vi "PID_controller_03.vi"() -> ()   [LabVIEW 2011]
uses:
  <vilib>/Platform/TimedLoop/XDataNode/nitl_modes.ctl
  <vilib>/Platform/TimedLoop/XDataNode/timing_clust.ctl
  <vilib>/Platform/TimedLoop/XDataNode/wakeup.ctl
  <vilib>/Platform/TimedLoop/XDataNode/XDataNode.xnode
  <vilib>/Platform/TimedLoop/XDataNode/XDNodeRunTimeDep.lvlib
panel:
  out "S00":dbl
  out "S10":dbl
  out "S20":dbl
  out "S11":dbl
  out "S01":dbl
  out "weight":dbl[](array[numeric])
  in  "# of points to watch":i32
  in  "alpha":dbl=-1.0
  out "t0":dbl
  out "error(t)":cluster{dbl, "Value":dbl}[](array[cluster])
  out "error out":errorcluster
  out "first":bool=TRUE
  out "P (torr)":string
  out "XY Graph":T1(graph)
  out "current value":dbl
  in  "stop":bool
  in  "Period (s)":dbl
  out "Process value":dbl
  out "derivative":dbl
  out "integral":dbl
  out "error":dbl
  out "Current angle (deg)":dbl
  in  "Kd":dbl
  in  "Ki":dbl
  in  "Kp":dbl
  out "Current P (torr)":dbl
  in  "Set Point (torr)":dbl
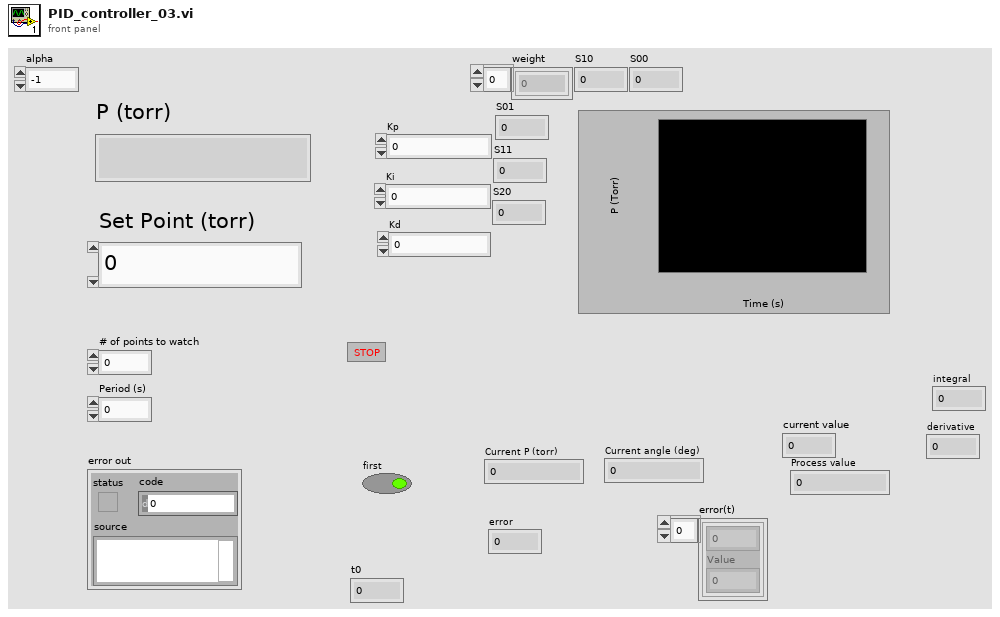
[diagram p1: front panel]
types:
  T1 = cluster{"Value":cluster{"element":dbl, "element":dbl}[]}[]
  T2 = typedef "XDNodeRunTimeDep.lvlib/nitl_modes.ctl" = enum32{"No Change", "Process missed periods, maintain original phase", "Discard missed periods, maintain original phase", "Process missed periods, ignore original phase", "Discard missed periods, ignore original phase"}
  T3 = typedef "XDNodeRunTimeDep.lvlib/timing_clust.ctl" = cluster{"Expected End [f-1]":u64, "Actual End [f-1]":u64, "Finished Late? [f-1]":bool, "Expected End [i-1]":u64, "Actual End [i-1]":u64, "Finished Late? [i-1]":bool, "Expected Start [i]":u64, "Actual Start [i]":u64, "Expected Start [f]":u64, "Actual Start [f]":u64, "Source Name":string, "Structure Name":string, "Period":i64, "Deadline":i64, "Offset":i64, "Start":i64, "Priority":i32, "Timeout":i32, "Mode":T2, "Wakeup Reason":T4, "Error":errorcluster, "Source Type":string, "Secondary Source Type":string, "Global End Time":u64, "Global Start Time":u64, "Frame Duration":u64, "Iteration Duration":u64, "Assigned CPU":i32, "I/O Scan Engine Mode":u32}
  T4 = typedef "XDNodeRunTimeDep.lvlib/wakeup.ctl" = enum32{"Normal", "Aborted", "Asynchronous wakeup", "Timing source error", "Timed loop error", "Timeout"}
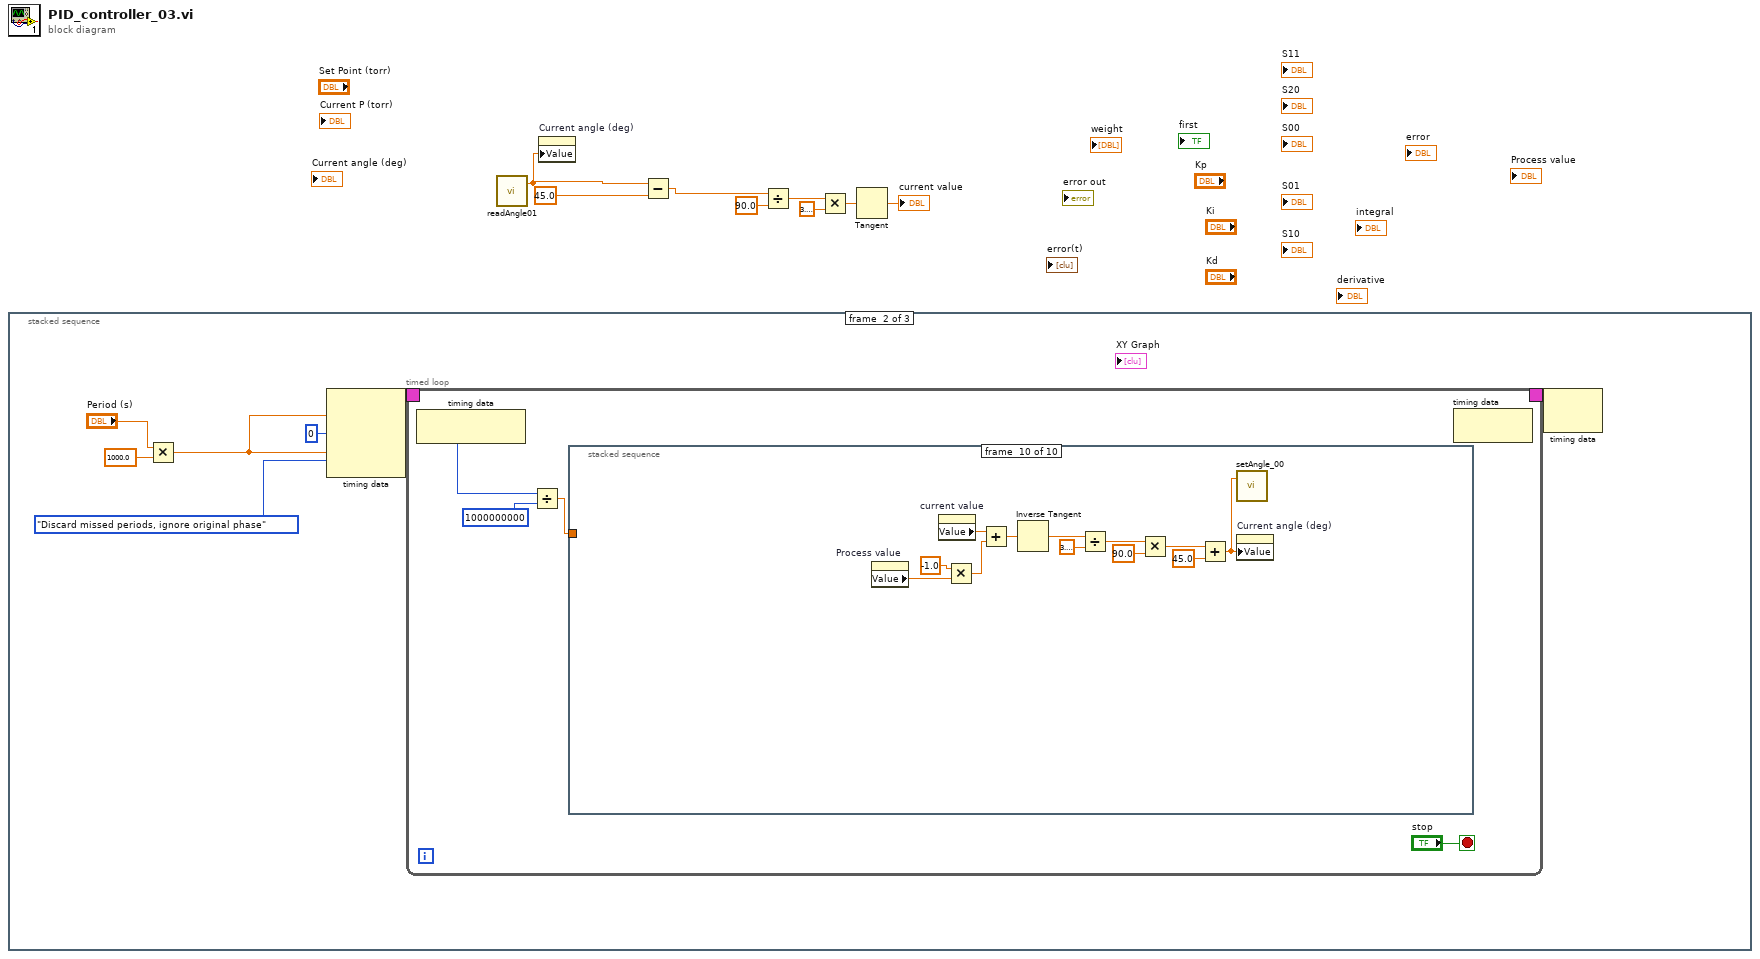
[diagram p0: block diagram]
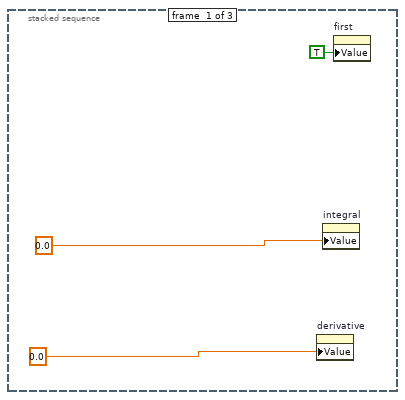
[diagram p2: hidden frame]
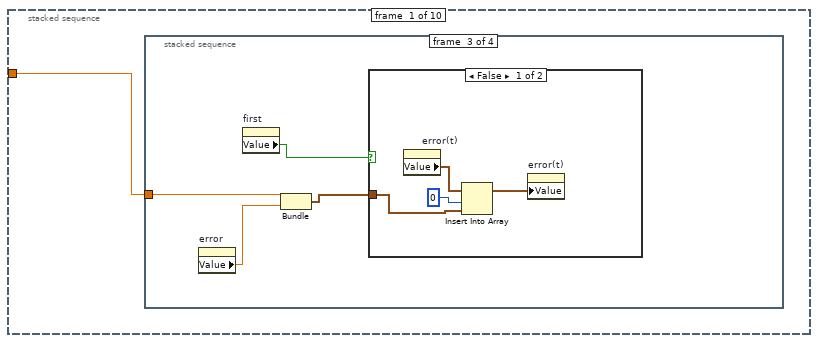
[diagram p3: hidden frame]
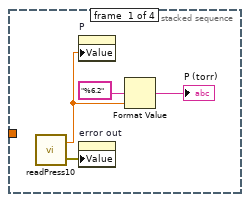
[diagram p4: hidden frame]
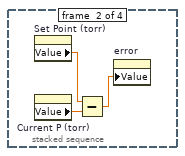
[diagram p5: hidden frame]
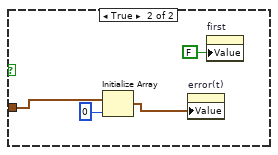
[diagram p6: hidden frame]
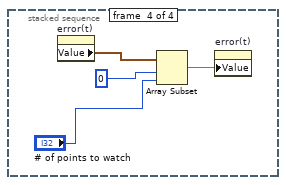
[diagram p7: hidden frame]
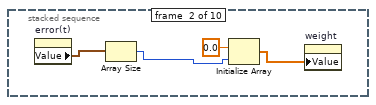
[diagram p8: hidden frame]
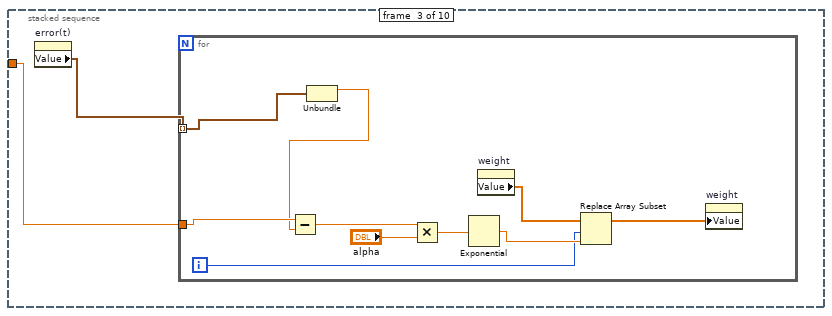
[diagram p9: hidden frame]
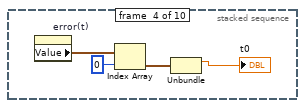
[diagram p10: hidden frame]
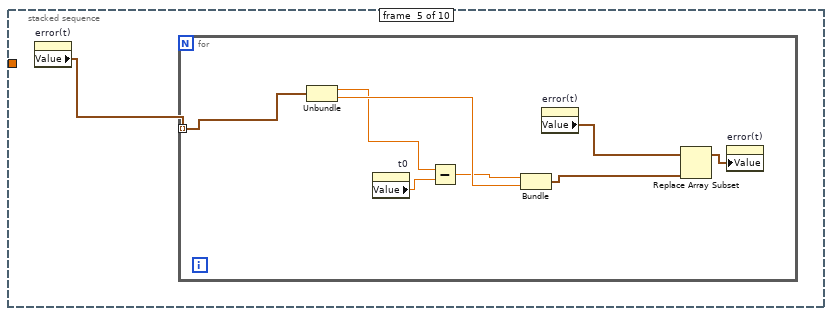
[diagram p11: hidden frame]
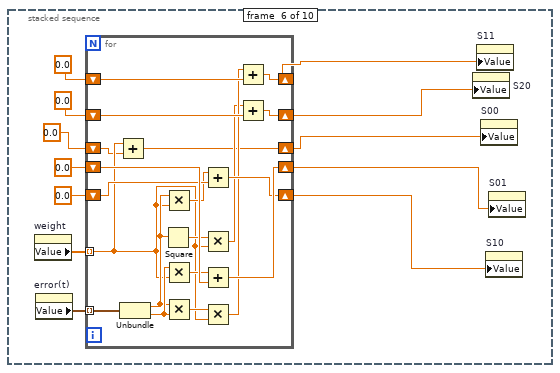
[diagram p12: hidden frame]
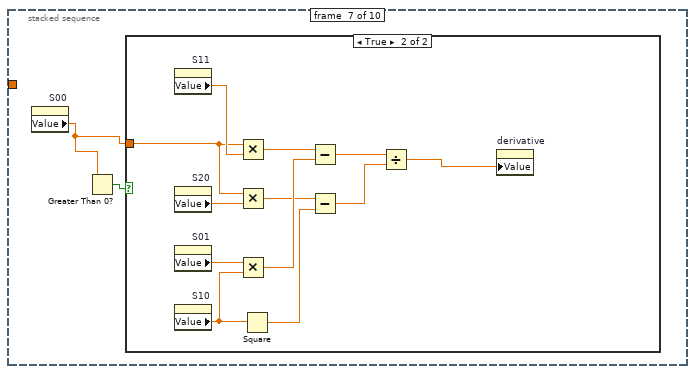
[diagram p13: hidden frame]
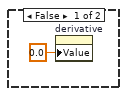
[diagram p14: hidden frame]
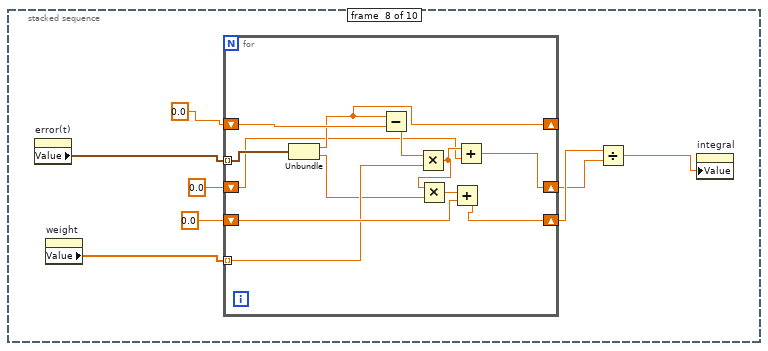
[diagram p15: hidden frame]
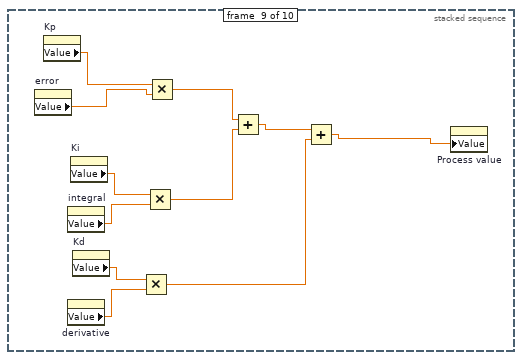
[diagram p16: hidden frame]
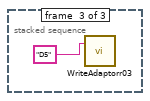
[diagram p17: hidden frame]
diagram:
  n1 = stacked-sequence {
    frame #0 {
      n2 = property on="derivative" class="DigNum (strict)"("Value"=0.0 ("derivative")) -> ()  [unwired: 2 in, 2 out]
      n3 = property on="integral" class="DigNum (strict)"("Value"=0.0 ("integral")) -> ()  [unwired: 2 in, 2 out]
      n4 = property on="first" class="Bool (strict)"("Value"=TRUE ("first")) -> ()  [unwired: 2 in, 2 out]
    }
    frame #1 {
      n5 = Multiply(x="Period (s)", y=1000.0) -> (x*y=w13:dbl)
      n6 = node-c288(w13, i64 0 ("Offset"), w13, nitl_modes."Discard missed periods, ignore original phase" ("Mode")) -> (w18:T3)
      n7 = timed-loop {
        timing: w18 -> [_]
        timing-out: [_] -> w17
        stop <- "stop" stop-if-true
        n8 = node-c288() -> (w21:i64)  [unwired: 1 in]
        n9 = Divide(x=w21, y=i64 1000000000) -> (x/y=w19:dbl)
        n10 = stacked-sequence {
          tunnel: w19 -> [w23 _ w51 _ _ _ _ _ _ _]
          frame #0 {
            n11 = stacked-sequence {
              tunnel: w23 -> [_ _ w33 _]
              frame #0 {
                n12 = call "readPress10.vi"() -> ("P"=w26:dbl, "error out"=w24:errorcluster)  [unwired: 1 in]
                n13 = property on="P" class="DigNum (strict)"("Value"=w26) -> ()  [unwired: 2 in, 2 out]
                n14 = property on="error out" class="Clust (strict)"("Value"=w24) -> ()  [unwired: 2 in, 2 out]
                n15 = Format Value(format string="%6.2", value (0)=w26) -> (output string=→"P (torr)":string)  [unwired: 1 in]
              }
              frame #1 {
                n16 = property on="Set Point (torr)" class="DigNum (strict)"() -> ("Value"=w29:dbl)  [unwired: 2 in, 2 out]
                n17 = property on="Current P (torr)" class="DigNum (strict)"() -> ("Value"=w30:dbl)  [unwired: 2 in, 2 out]
                n18 = Subtract(x=w29, y=w30) -> (x-y=w28:dbl)
                n19 = property on="error" class="DigNum (strict)"("Value"=w28) -> ()  [unwired: 2 in, 2 out]
              }
              frame #2 {
                n20 = property on="error" class="DigNum (strict)"() -> ("Value"=w32:dbl)  [unwired: 2 in, 2 out]
                n21 = property on="first" class="Bool (strict)"() -> ("Value"=w34:bool)  [unwired: 2 in, 2 out]
                n22 = Bundle(w33, "Value"=w32) -> (w31:cluster{dbl, "Value":dbl})  [unwired: 1 in]
                n23 = case shown="False" w34 {
                  tunnel: w31 -> [w35 w41]
                  frame False {
                    n24 = property on="error(t)" class="Arr (strict)"() -> ("Value"=w36:cluster{dbl, "Value":dbl}[])  [unwired: 2 in, 2 out]
                    n25 = Insert Into Array(array=w36, index=0, new element=w35) -> (w38:cluster{dbl, "Value":dbl}[])
                    n26 = property on="error(t)" class="Arr (strict)"("Value"=w38) -> ()  [unwired: 2 in, 2 out]
                  }
                  frame True {
                    n27 = Initialize Array(w41, 0 ("dimension size")) -> (w39:cluster{dbl, "Value":dbl}[])
                    n28 = property on="error(t)" class="Arr (strict)"("Value"=w39) -> ()  [unwired: 2 in, 2 out]
                    n29 = property on="first" class="Bool (strict)"("Value"=FALSE ("first")) -> ()  [unwired: 2 in, 2 out]
                  }
                }
              }
              frame #3 {
                n30 = property on="error(t)" class="Arr (strict)"() -> ("Value"=w44:cluster{dbl, "Value":dbl}[])  [unwired: 2 in, 2 out]
                n31 = Array Subset(array=w44, index=0, length="# of points to watch") -> (w46:cluster{dbl, "Value":dbl}[])
                n32 = property on="error(t)" class="Arr (strict)"("Value"=w46) -> ()  [unwired: 2 in, 2 out]
              }
            }
          }
          frame #1 {
            n33 = property on="error(t)" class="Arr (strict)"() -> ("Value"=w50:cluster{dbl, "Value":dbl}[])  [unwired: 2 in, 2 out]
            n34 = Array Size(array=w50) -> (size(s)=w48:i32)
            n35 = Initialize Array(0.0 ("element"), w48) -> (w47:dbl[])
            n36 = property on="weight" class="Arr (strict)"("Value"=w47) -> ()  [unwired: 2 in, 2 out]
          }
          frame #2 {
            n37 = property on="error(t)" class="Arr (strict)"() -> ("Value"=w52:cluster{dbl, "Value":dbl}[])  [unwired: 2 in, 2 out]
            n38 = for {
              tunnel: w52 -> [w62] mode=indexing
              tunnel: w51 -> [w59]
              i -> [w54]
              n39 = Unbundle(w62) -> (w58:dbl)  [unwired: 1 out]
              n40 = Subtract(x=w59, y=w58) -> (x-y=w57:dbl)
              n41 = Multiply(x=w57, y="alpha") -> (x*y=w60:dbl)
              n42 = Exponential(1:w60) -> (0:w56:dbl)
              n43 = property on="weight" class="Arr (strict)"() -> ("Value"=w55:dbl[])  [unwired: 2 in, 2 out]
              n44 = Replace Array Subset(array=w55, new element=w56, index=w54) -> (w53:dbl[])
              n45 = property on="weight" class="Arr (strict)"("Value"=w53) -> ()  [unwired: 2 in, 2 out]
            }
          }
          frame #3 {
            n46 = property on="error(t)" class="Arr (strict)"() -> ("Value"=w66:cluster{dbl, "Value":dbl}[])  [unwired: 2 in, 2 out]
            n47 = Index Array(array=w66, index=0) -> (element=w64:cluster{dbl, "Value":dbl})
            n48 = Unbundle(w64) -> (→"t0":dbl)  [unwired: 1 out]
          }
          frame #4 {
            n49 = property on="error(t)" class="Arr (strict)"() -> ("Value"=w67:cluster{dbl, "Value":dbl}[])  [unwired: 2 in, 2 out]
            n50 = for {
              tunnel: w67 -> [w72] mode=indexing
              n51 = Unbundle(w72) -> (w69:dbl, "Value"=w74:dbl)
              n52 = property on="t0" class="DigNum (strict)"() -> ("Value"=w75:dbl)  [unwired: 2 in, 2 out]
              n53 = Subtract(x=w69, y=w75) -> (x-y=w70:dbl)
              n54 = Bundle(w70, "Value"=w74) -> (w68:cluster{dbl, "Value":dbl})  [unwired: 1 in]
              n55 = property on="error(t)" class="Arr (strict)"() -> ("Value"=w73:cluster{dbl, "Value":dbl}[])  [unwired: 2 in, 2 out]
              n56 = Replace Array Subset(array=w73, new element=w68) -> (w71:cluster{dbl, "Value":dbl}[])  [unwired: 1 in]
              n57 = property on="error(t)" class="Arr (strict)"("Value"=w71) -> ()  [unwired: 2 in, 2 out]
            }
          }
          frame #5 {
            n58 = property on="weight" class="Arr (strict)"() -> ("Value"=w82:dbl[])  [unwired: 2 in, 2 out]
            n59 = property on="error(t)" class="Arr (strict)"() -> ("Value"=w87:cluster{dbl, "Value":dbl}[])  [unwired: 2 in, 2 out]
            n60 = for {
              tunnel: w87 -> [w103] mode=indexing
              shift-right: [w104] -> w77
              shift-left: 0.0 -> [w107]
              shift-right: [w100] -> w80
              shift-left: 0.0 -> [w106]
              shift-right: [w99] -> w79
              shift-left: 0.0 -> [w105]
              shift-right: [w101] -> w76
              shift-left: 0.0 -> [w102]
              tunnel: w82 -> [w90] mode=indexing
              shift-right: [w88] -> w78
              shift-left: 0.0 -> [w89]
              n61 = Add(x=w90, y=w89) -> (x+y=w88:dbl)
              n62 = Unbundle(w103) -> (w92:dbl, "Value"=w98:dbl)
              n63 = Square(x=w92) -> (x^2=w94:dbl)
              n64 = Multiply(x=w92, y=w90) -> (x*y=w91:dbl)
              n65 = Multiply(x=w98, y=w90) -> (x*y=w97:dbl)
              n66 = Multiply(x=w92, y=w98) -> (x*y=w96:dbl)
              n67 = Add(x=w91, y=w102) -> (x+y=w101:dbl)
              n68 = Multiply(x=w94, y=w90) -> (x*y=w93:dbl)
              n69 = Add(x=w97, y=w107) -> (x+y=w104:dbl)
              n70 = Multiply(x=w96, y=w90) -> (x*y=w95:dbl)
              n71 = Add(x=w95, y=w106) -> (x+y=w100:dbl)
              n72 = Add(x=w93, y=w105) -> (x+y=w99:dbl)
            }
            n73 = property on="S20" class="DigNum (strict)"("Value"=w79) -> ()  [unwired: 2 in, 2 out]
            n74 = property on="S11" class="DigNum (strict)"("Value"=w80) -> ()  [unwired: 2 in, 2 out]
            n75 = property on="S00" class="DigNum (strict)"("Value"=w78) -> ()  [unwired: 2 in, 2 out]
            n76 = property on="S10" class="DigNum (strict)"("Value"=w76) -> ()  [unwired: 2 in, 2 out]
            n77 = property on="S01" class="DigNum (strict)"("Value"=w77) -> ()  [unwired: 2 in, 2 out]
          }
          frame #6 {
            n78 = property on="S00" class="DigNum (strict)"() -> ("Value"=w108:dbl)  [unwired: 2 in, 2 out]
            n79 = Greater Than 0?(x=w108) -> (x > 0?=w109:bool)
            n80 = case shown="True" w109 {
              tunnel: w108 -> [_ w113]
              frame False {
                n81 = property on="derivative" class="DigNum (strict)"("Value"=0.0 ("derivative")) -> ()  [unwired: 2 in, 2 out]
              }
              frame True {
                n82 = property on="S11" class="DigNum (strict)"() -> ("Value"=w115:dbl)  [unwired: 2 in, 2 out]
                n83 = property on="S20" class="DigNum (strict)"() -> ("Value"=w114:dbl)  [unwired: 2 in, 2 out]
                n84 = property on="S01" class="DigNum (strict)"() -> ("Value"=w112:dbl)  [unwired: 2 in, 2 out]
                n85 = property on="S10" class="DigNum (strict)"() -> ("Value"=w116:dbl)  [unwired: 2 in, 2 out]
                n86 = Multiply(x=w113, y=w115) -> (x*y=w122:dbl)
                n87 = Multiply(x=w113, y=w114) -> (x*y=w120:dbl)
                n88 = Multiply(x=w112, y=w116) -> (x*y=w121:dbl)
                n89 = Square(x=w116) -> (x^2=w119:dbl)
                n90 = Subtract(x=w122, y=w121) -> (x-y=w118:dbl)
                n91 = Subtract(x=w120, y=w119) -> (x-y=w117:dbl)
                n92 = Divide(x=w118, y=w117) -> (x/y=w111:dbl)
                n93 = property on="derivative" class="DigNum (strict)"("Value"=w111) -> ()  [unwired: 2 in, 2 out]
              }
            }
          }
          frame #7 {
            n94 = property on="error(t)" class="Arr (strict)"() -> ("Value"=w130:cluster{dbl, "Value":dbl}[])  [unwired: 2 in, 2 out]
            n95 = property on="weight" class="Arr (strict)"() -> ("Value"=w128:dbl[])  [unwired: 2 in, 2 out]
            n96 = for {
              tunnel: w130 -> [w142] mode=indexing
              shift-right: [w140] -> _
              shift-left: 0.0 -> [w141]
              tunnel: w128 -> [w135] mode=indexing
              shift-right: [w136] -> w125
              shift-left: 0.0 -> [w137]
              shift-right: [w132] -> w124
              shift-left: 0.0 -> [w131]
              n97 = Unbundle(w142) -> (w140:dbl, "Value"=w134:dbl)
              n98 = Subtract(x=w140, y=w141) -> (x-y=w139:dbl)
              n99 = Multiply(x=w139, y=w135) -> (x*y=w133:dbl)
              n100 = Multiply(x=w133, y=w134) -> (x*y=w138:dbl)
              n101 = Add(x=w138, y=w137) -> (x+y=w136:dbl)
              n102 = Add(x=w133, y=w131) -> (x+y=w132:dbl)
            }
            n103 = Divide(x=w125, y=w124) -> (x/y=w123:dbl)
            n104 = property on="integral" class="DigNum (strict)"("Value"=w123) -> ()  [unwired: 2 in, 2 out]
          }
          frame #8 {
            n105 = property on="error" class="DigNum (strict)"() -> ("Value"=w153:dbl)  [unwired: 2 in, 2 out]
            n106 = property on="Kp" class="DigNum (strict)"() -> ("Value"=w152:dbl)  [unwired: 2 in, 2 out]
            n107 = property on="integral" class="DigNum (strict)"() -> ("Value"=w150:dbl)  [unwired: 2 in, 2 out]
            n108 = property on="derivative" class="DigNum (strict)"() -> ("Value"=w148:dbl)  [unwired: 2 in, 2 out]
            n109 = property on="Ki" class="DigNum (strict)"() -> ("Value"=w151:dbl)  [unwired: 2 in, 2 out]
            n110 = property on="Kd" class="DigNum (strict)"() -> ("Value"=w149:dbl)  [unwired: 2 in, 2 out]
            n111 = Multiply(x=w149, y=w148) -> (x*y=w145:dbl)
            n112 = Multiply(x=w151, y=w150) -> (x*y=w146:dbl)
            n113 = Multiply(x=w152, y=w153) -> (x*y=w147:dbl)
            n114 = Add(x=w147, y=w146) -> (x+y=w144:dbl)
            n115 = Add(x=w144, y=w145) -> (x+y=w143:dbl)
            n116 = property on="Process value" class="DigNum (strict)"("Value"=w143) -> ()  [unwired: 2 in, 2 out]
          }
          frame #9 {
            n117 = property on="Process value" class="DigNum (strict)"() -> ("Value"=w163:dbl)  [unwired: 2 in, 2 out]
            n118 = property on="current value" class="DigNum (strict)"() -> ("Value"=w156:dbl)  [unwired: 2 in, 2 out]
            n119 = Multiply(x=-1.0, y=w163) -> (x*y=w164:dbl)
            n120 = Add(x=w156, y=w164) -> (x+y=w155:dbl)
            n121 = Inverse Tangent(1:w155) -> (0:w162:dbl)
            n122 = Divide(x=w162, y=3.141592653589793) -> (x/y=w160:dbl)
            n123 = Multiply(x=w160, y=90.0) -> (x*y=w158:dbl)
            n124 = Add(x=w158, y=45.0) -> (x+y=w154:dbl)
            n125 = call "setAngle_00.vi"("Angle (deg)"=w154) -> ()  [unwired: 1 in, 1 out]
            n126 = property on="Current angle (deg)" class="DigNum (strict)"("Value"=w154) -> ()  [unwired: 2 in, 2 out]
          }
        }
        n127 = node-c288() -> ()  [unwired: 1 in, 1 out]
      }
      n128 = node-c288(w17) -> ()  [unwired: 1 out]
    }
    frame #2 {
      n129 = call "WriteAdaptorr03.vi"("string to write"="D5") -> ()  [unwired: 1 in, 1 out]
    }
  }
  n130 = call "readAngle01.vi"() -> ("angle"=w2:dbl)  [unwired: 1 in, 1 out]
  n131 = property on="Current angle (deg)" class="DigNum (strict)"("Value"=w2) -> ()  [unwired: 2 in, 2 out]
  n132 = Subtract(x=w2, y=45.0) -> (x-y=w8:dbl)
  n133 = Divide(x=w8, y=90.0) -> (x/y=w4:dbl)
  n134 = Multiply(x=w4, y=3.141592653589793) -> (x*y=w6:dbl)
  n135 = Tangent(1:w6) -> (0:→"current value":dbl)
